vi "GET Data.vi"() -> (0 "Data":dbl[][](array[numeric]))   [LabVIEW 2013]
uses:
  Action.ctl
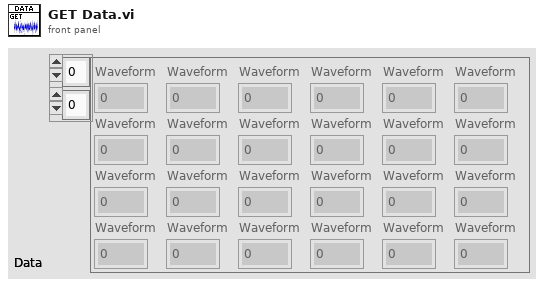
[diagram p1: front panel]
types:
  T1 = typedef "Action.ctl" = enum16{"GET", "PUT", "DELETE"}
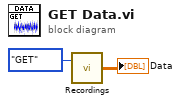
[diagram p0: block diagram]
diagram:
  n1 = call "Recordings.vi"("Action"=Action."GET") -> ("Data Out"=→"Data":dbl[][])  [unwired: 1 in]
